vi "IMAQDevice.ProcCases.vi"(0 "i ref in":refnum<vi>, 1 "selector":string, 2 "Data":T1, 3 "call cluster":T2={"Object"="", "Selector"="", "CallType"=enum."synchronous", "Async Object"="", "Async Selector"="", "Data Descriptor"="", "Data"=[], "Error #"=0, "Expire"=0}, 5 "error in (no error)":errorcluster) -> (14 "i ref out":refnum<vi>, 17 "answer cluster":T2={"Object"="", "Selector"="", "CallType"=enum."synchronous", "Async Object"="", "Async Selector"="", "Data Descriptor"="", "Data"=[], "Error #"=0, "Expire"=0}, 19 "error out":errorcluster)   [LabVIEW 2014, in "IMAQDevice.lvlib"]
doc: "This method is called by a process from within the default case in the event loop. The methods of a class that are linked to events will be called from THIS method. Add your code here."
uses:
  IMAQDevice.lvlib
  CSCore/CSApplicationBaseClasses/DeviceBase/DeviceBase.lvlib
  CSCore/BaseProcess/BaseProcess.lvlib
  CSCore/CSSystem/CoreLib/CoreLib.lvlib
  CSCore/CSSystem/CoreLib/CoreLib.string 2 byte array.vi
  CSCore/CSSystem/CoreLib/CoreLib.byte array 2 short.vi
  CSCore/CSSystem/CoreLib/CoreLib.byte array 2 int.vi
  CSCore/CSSystem/CoreLib/CoreLib.int 2 byte array.vi
  CSCore/CSSystem/CoreLib/CoreLib.double 2 byte array.vi
  CSCore/BaseProcess/BaseProcess.descriptor string definition.ctl
  CSlibraries-extern/DimLVEvent/LVDimInterface/LVDimInterface.lvlib
  CSCore/CSSystem/CoreDefs/CoreDefs.call_type.ctl
  CSCore/CSSystem/CoreDefs/CoreDefs.rawDataType.ctl
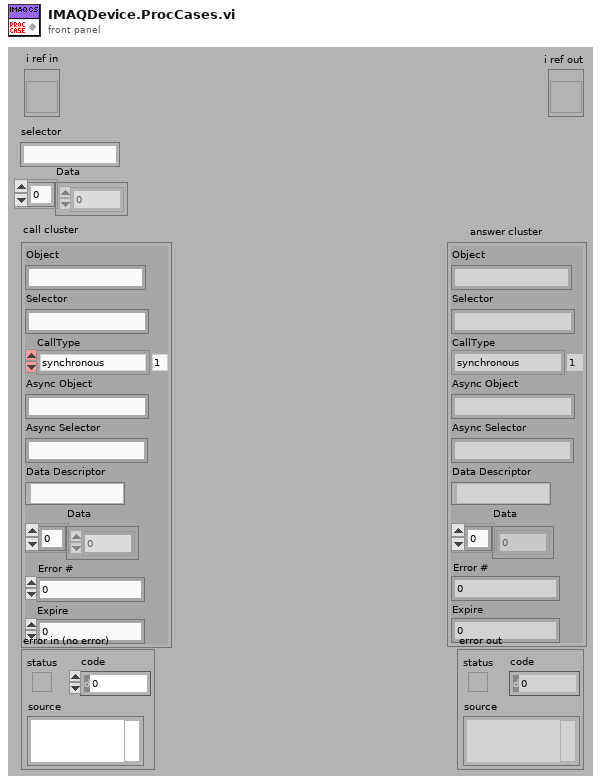
[diagram p1: front panel]
types:
  T1 = typedef "CoreDefs.rawDataType.ctl" = i8[]
  T2 = typedef "CoreDefs.call_type.ctl" = cluster{"Object":string, "Selector":string, "CallType":enum16{"simple", "synchronous", "asynchronous"}, "Async Object":string, "Async Selector":string, "Data Descriptor":T3, "Data":T1, "Error #":i32, "Expire":u32}
  T3 = typedef "BaseProcess.lvlib/BaseProcess.descriptor string definition.ctl" = string
  T4 = typedef "IMAQDevice.lvlib/IMAQDevice.i attribute.ctl" = cluster{"HGF_IMAQ.lvlib:HGF_IMAQDevice.lvclass":refnum<class "HGF_IMAQDevice.lvclass">, "Image":T5, "TimeStampID":i32, "Image IDs":i32[], "NumberOfImagesID":i32, "JPEG?":bool, "JPEGID":i32, "JPEG_ImageID":i32, "TriggerModeID":i32, "OffsetFromLeft":i32, "OffsetFromTop":i32, "HorizontalPixelPerMm":dbl, "VerticalPixelPerMm":dbl, "Grid":cluster{"1":cluster{i32, i32}, "2":cluster{i32, i32}, "3":cluster{i32, i32}, "4":cluster{i32, i32}}, "GridR":cluster{"1":cluster{dbl, dbl}, "2":cluster{dbl, dbl}, "3":cluster{dbl, dbl}, "4":cluster{dbl, dbl}}, "CameraTypeID":i32, "CameraInfos":cluster{"Camera Name-Array":string[], "own Camera Type":string}, "TakeMeasurement?":bool, "TriggerArmedID":i32, "Mirroring":i16, "Rotation":dbl}
  T5 = typedef "IMAQ Image.ctl" = refnum<image>
  T6 = cluster{"1":cluster{i32, i32}, "2":cluster{i32, i32}, "3":cluster{i32, i32}, "4":cluster{i32, i32}}
  T7 = cluster{"1":cluster{dbl, dbl}, "2":cluster{dbl, dbl}, "3":cluster{dbl, dbl}, "4":cluster{dbl, dbl}}
  T8 = cluster{"Grid":cluster{"1":cluster{i32, i32}, "2":cluster{i32, i32}, "3":cluster{i32, i32}, "4":cluster{i32, i32}}, "GridR":cluster{"1":cluster{dbl, dbl}, "2":cluster{dbl, dbl}, "3":cluster{dbl, dbl}, "4":cluster{dbl, dbl}}}
  T9 = cluster{"Camera Name-Array":string[], "own Camera Type":string}
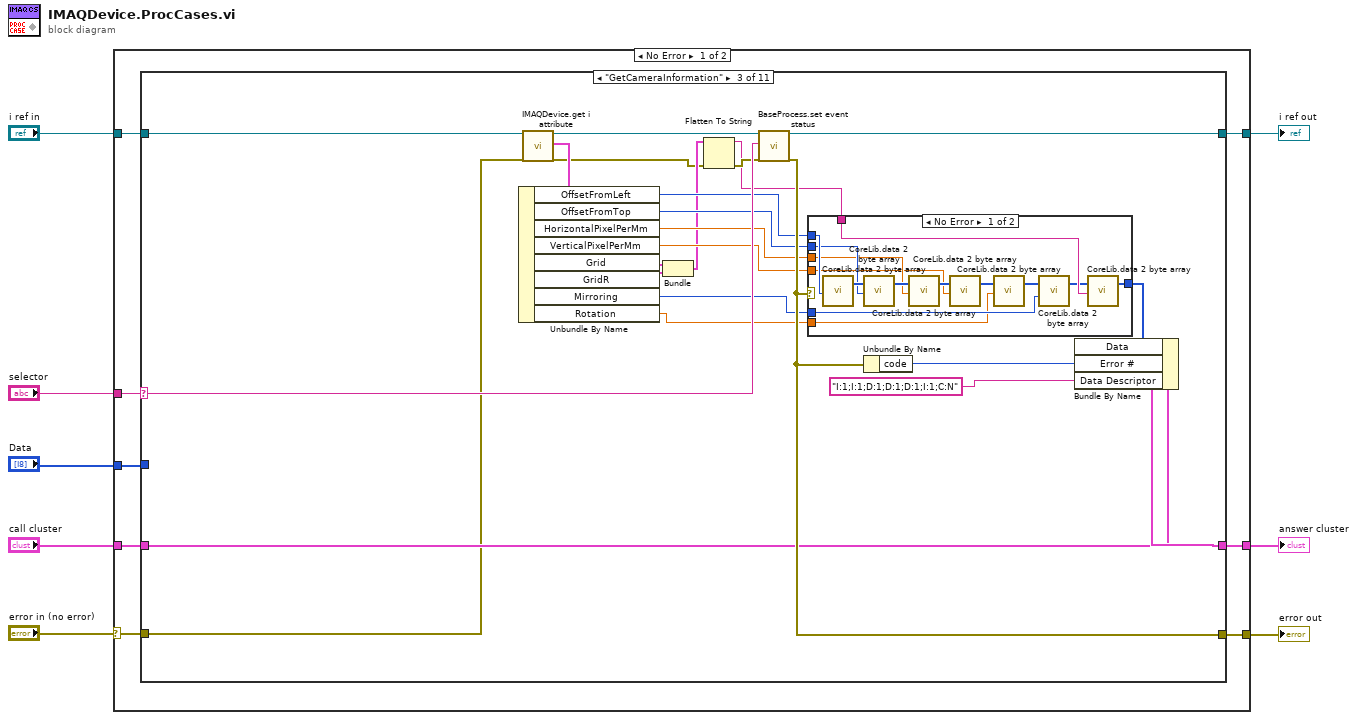
[diagram p0: block diagram]
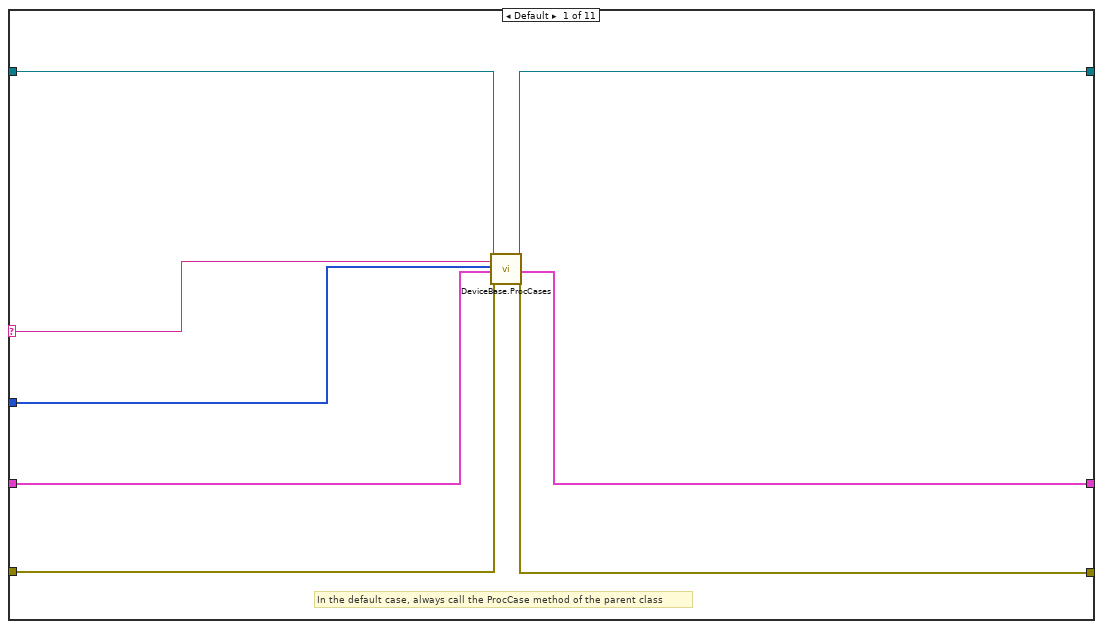
[diagram p2: hidden frame]
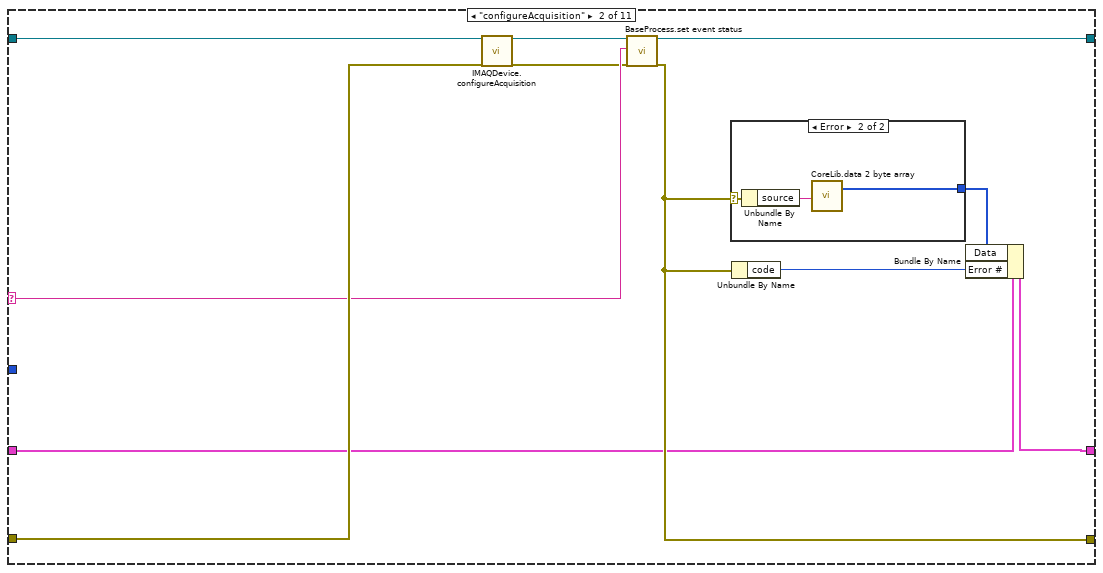
[diagram p3: hidden frame]
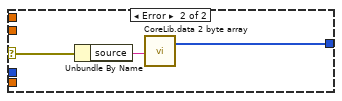
[diagram p5: hidden frame]
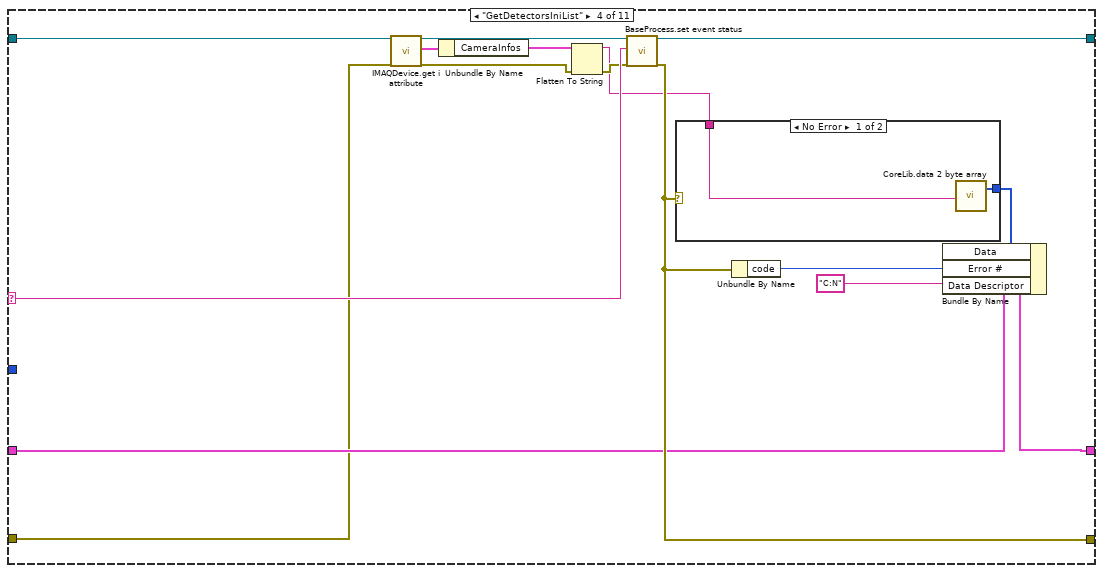
[diagram p6: hidden frame]
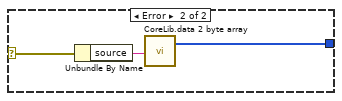
[diagram p7: hidden frame]
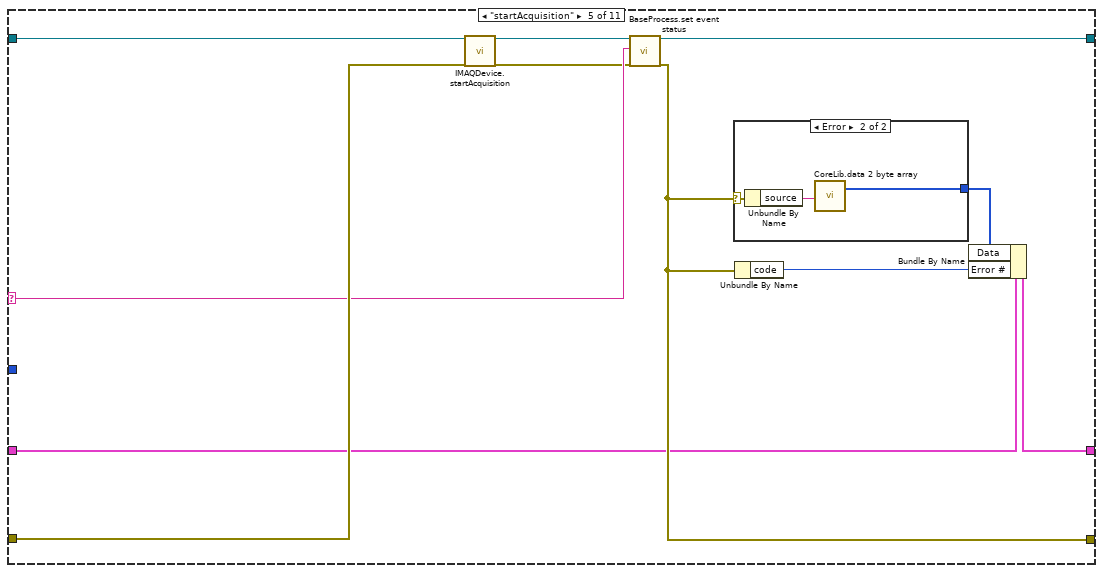
[diagram p8: hidden frame]
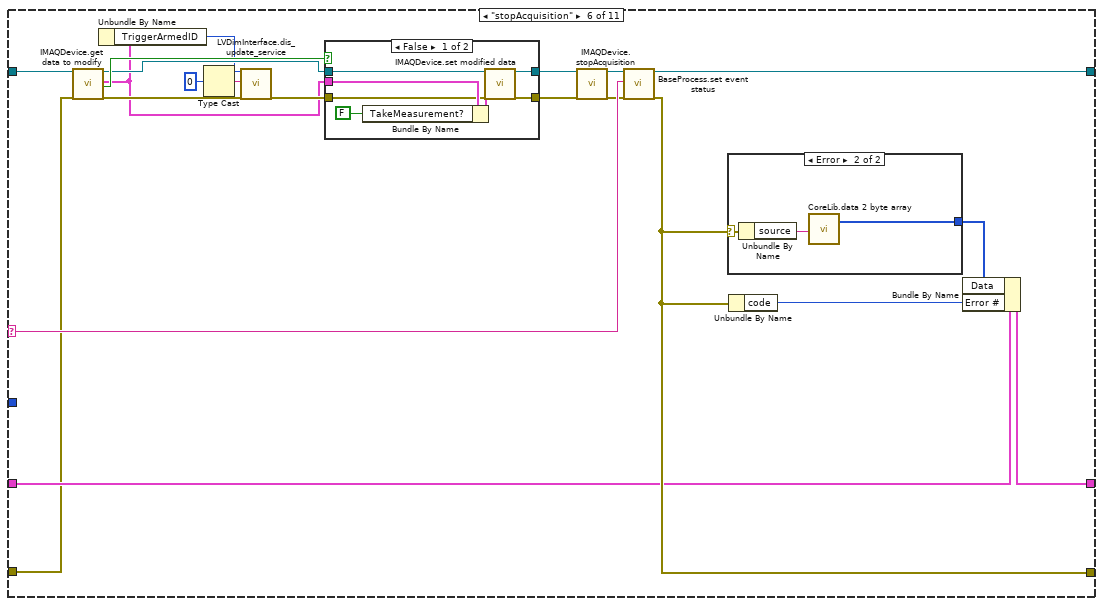
[diagram p10: hidden frame]
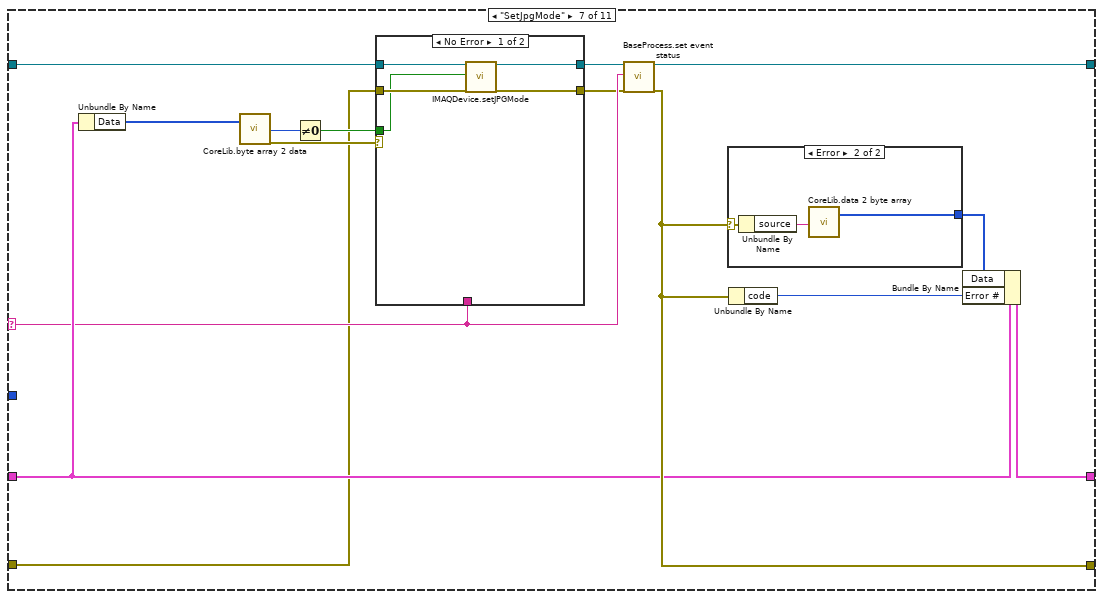
[diagram p13: hidden frame]
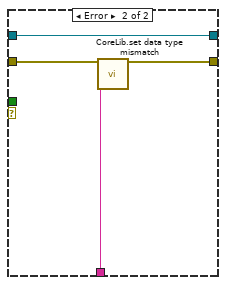
[diagram p14: hidden frame]
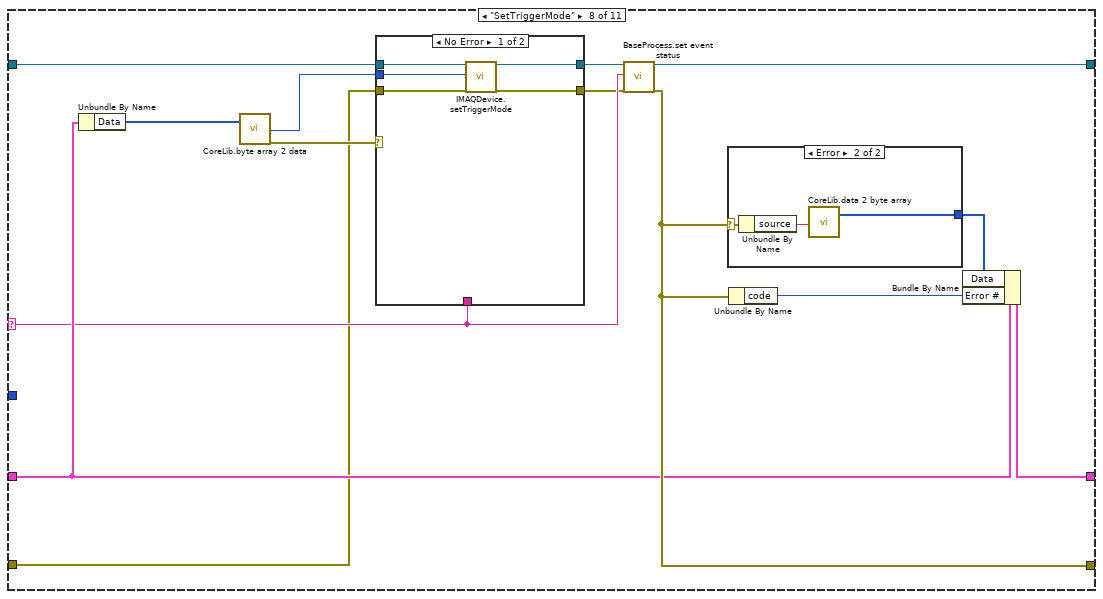
[diagram p16: hidden frame]
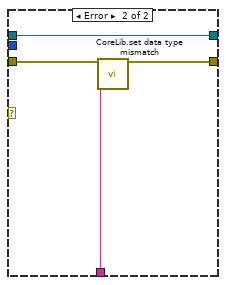
[diagram p17: hidden frame]
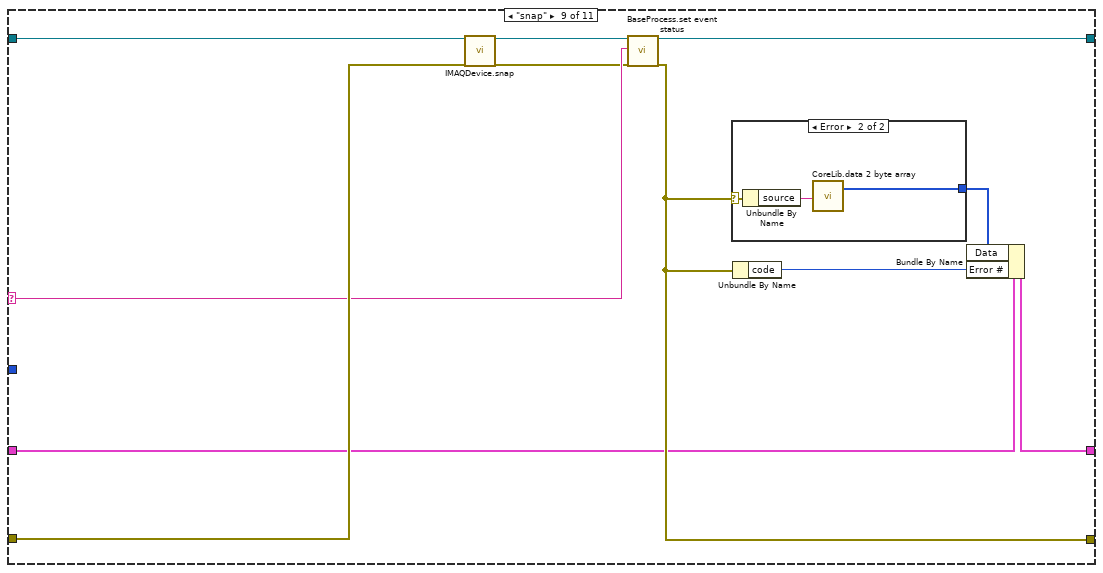
[diagram p19: hidden frame]
diagram:
  n1 = case shown="No Error" "error in (no error)" {
    selector: "error in (no error)" -> [w9 w260]
    tunnel: "selector" -> [w16 _]
    tunnel: [w15 w261] -> w7
    tunnel: "Data" -> [w14 _]
    tunnel: "call cluster" -> [w13 w261]
    tunnel: "i ref in" -> [w12 w262]
    tunnel: [w11 w262] -> w3
    tunnel: [w10 w260] -> w2
    frame No Error {
      n2 = case shown="\"GetCameraInformation\"" w16 {
        selector: w16 -> [w19 w31 w60 w93 w107 w133 w154 w181 w207 w231 w252]
        tunnel: w14 -> [w17 _ _ _ _ _ _ _ _ _ _]
        tunnel: w12 -> [w18 w35 w53 w86 w111 w125 w150 w178 w211 w226 w256]
        tunnel: [w24 w29 w59 w92 w102 w128 w158 w184 w202 w230 w249] -> w11
        tunnel: w13 -> [w20 w25 w56 w89 w103 w129 w155 w182 w203 w227 w246]
        tunnel: [w21 w26 w57 w90 w104 w130 w159 w185 w204 w228 w247] -> w15
        tunnel: w9 -> [w23 w34 w55 w88 w110 w123 w151 w179 w210 w225 w255]
        tunnel: [w22 w27 w58 w91 w105 w131 w160 w186 w205 w229 w248] -> w10
        frame Default {
          # "In the default case, always call the ProcCase method of the parent class"
          n3 = call "DeviceBase.ProcCases.vi"("i ref in"=w18, "selector"=w19, "Data"=w17, "call cluster"=w20, "error in (no error)"=w23) -> ("i ref out"=w24:refnum<vi>, "answer cluster"=w21:T2, "error out"=w22:errorcluster)  [unwired: 12 in]
        }
        frame "configureAcquisition" {
          n4 = call "IMAQDevice.configureAcquisition.vi"("i ref in"=w35, "error in (no error)"=w34) -> ("i ref out"=w28:refnum<vi>, "error out"=w30:errorcluster)  [unwired: 16 in]
          n5 = call "BaseProcess.set event status.vi"("i ref in"=w28, "EventStatus"=w31, "error in (no error)"=w30) -> ("i ref out"=w29:refnum<vi>, "error out"=w27:errorcluster)  [unwired: 14 in, 1 out]
          n6 = case shown="Error" w27 {
            selector: w27 -> [_ w38]
            tunnel: [_ w36] -> w32
            frame No Error {
            }
            frame Error {
              n7 = Unbundle By Name(w38) -> ("source"=w37:string)
              n8 = call-poly "CoreLib.data 2 byte array.vi"("string"=w37) -> ("byteArray out"=w36:T1)  [unwired: 18 in]
            }
          }
          n9 = Unbundle By Name(w27) -> ("code"=w33:i32)
          n10 = Bundle By Name(cluster=w25, "Data"=w32, "Error #"=w33) -> (w26:T2)
        }
        frame "GetCameraInformation" {
          n11 = call "IMAQDevice.get i attribute.vi"("i ref in"=w53, "error in (no error)"=w55) -> ("i ref out"=w54:refnum<vi>, "i attribute"=w52:T4, "error out"=w44:errorcluster)  [unwired: 15 in]
          n12 = Unbundle By Name(w52) -> ("OffsetFromLeft"=w51:i32, "OffsetFromTop"=w50:i32, "HorizontalPixelPerMm"=w49:dbl, "VerticalPixelPerMm"=w48:dbl, "Grid"=w47:T6, "GridR"=w46:T7, "Mirroring"=w40:i16, "Rotation"=w39:dbl)
          n13 = Bundle("Grid"=w47, "GridR"=w46) -> (w45:T8)  [unwired: 1 in]
          n14 = Flatten To String(anything=w45, error in (no error)=w44) -> (data string=w42:string, error out=w43:errorcluster)  [unwired: 2 in, 1 out]
          n15 = call "BaseProcess.set event status.vi"("i ref in"=w54, "EventStatus"=w60, "error in (no error)"=w43) -> ("i ref out"=w59:refnum<vi>, "error out"=w58:errorcluster)  [unwired: 14 in, 1 out]
          n16 = case shown="No Error" w58 {
            selector: w58 -> [_ w79]
            tunnel: [w69 w77] -> w61
            tunnel: w51 -> [w76 _]
            tunnel: w50 -> [w74 _]
            tunnel: w49 -> [w71 _]
            tunnel: w48 -> [w70 _]
            tunnel: w42 -> [w68 _]
            tunnel: w40 -> [w66 _]
            tunnel: w39 -> [w63 _]
            frame No Error {
              n17 = call-poly "CoreLib.data 2 byte array.vi"("i32"=w76) -> ("byteArray out"=w75:T1)  [unwired: 18 in]
              n18 = call-poly "CoreLib.data 2 byte array.vi"("byteArray"=w75, "i32"=w74) -> ("byteArray out"=w73:T1)  [unwired: 17 in]
              n19 = call-poly "CoreLib.data 2 byte array.vi"("byteArray"=w73, "f64"=w71) -> ("byteArray out"=w72:T1)  [unwired: 17 in]
              n20 = call-poly "CoreLib.data 2 byte array.vi"("byteArray"=w72, "f64"=w70) -> ("byteArray out"=w65:T1)  [unwired: 17 in]
              n21 = call-poly "CoreLib.data 2 byte array.vi"("byteArray"=w65, "f64"=w63) -> ("byteArray out"=w64:T1)  [unwired: 17 in]
              n22 = call-poly "CoreLib.data 2 byte array.vi"("byteArray"=w64, "i32"=w66) -> ("byteArray out"=w67:T1)  [unwired: 17 in]
              n23 = call-poly "CoreLib.data 2 byte array.vi"("byteArray"=w67, "string"=w68) -> ("byteArray out"=w69:T1)  [unwired: 17 in]
            }
            frame Error {
              n24 = Unbundle By Name(w79) -> ("source"=w78:string)
              n25 = call-poly "CoreLib.data 2 byte array.vi"("string"=w78) -> ("byteArray out"=w77:T1)  [unwired: 18 in]
            }
          }
          n26 = Unbundle By Name(w58) -> ("code"=w62:i32)
          n27 = Bundle By Name(cluster=w56, "Data"=w61, "Error #"=w62, "Data Descriptor"=T3 "I:1;I:1;D:1;D:1;D:1;I:1;C:N") -> (w57:T2)
        }
        frame "GetDetectorsIniList" {
          n28 = call "IMAQDevice.get i attribute.vi"("i ref in"=w86, "error in (no error)"=w88) -> ("i ref out"=w87:refnum<vi>, "i attribute"=w85:T4, "error out"=w84:errorcluster)  [unwired: 15 in]
          n29 = Unbundle By Name(w85) -> ("CameraInfos"=w80:T9)
          n30 = Flatten To String(anything=w80, error in (no error)=w84) -> (data string=w82:string, error out=w83:errorcluster)  [unwired: 2 in, 1 out]
          n31 = call "BaseProcess.set event status.vi"("i ref in"=w87, "EventStatus"=w93, "error in (no error)"=w83) -> ("i ref out"=w92:refnum<vi>, "error out"=w91:errorcluster)  [unwired: 14 in, 1 out]
          n32 = case shown="No Error" w91 {
            selector: w91 -> [_ w100]
            tunnel: [w97 w98] -> w94
            tunnel: w82 -> [w96 _]
            frame No Error {
              n33 = call-poly "CoreLib.data 2 byte array.vi"("string"=w96) -> ("byteArray out"=w97:T1)  [unwired: 18 in]
            }
            frame Error {
              n34 = Unbundle By Name(w100) -> ("source"=w99:string)
              n35 = call-poly "CoreLib.data 2 byte array.vi"("string"=w99) -> ("byteArray out"=w98:T1)  [unwired: 18 in]
            }
          }
          n36 = Unbundle By Name(w91) -> ("code"=w95:i32)
          n37 = Bundle By Name(cluster=w89, "Data"=w94, "Error #"=w95, "Data Descriptor"=T3 "C:N") -> (w90:T2)
        }
        frame "startAcquisition" {
          n38 = call "IMAQDevice.startAcquisition.vi"("i ref in"=w111, "error in (no error)"=w110) -> ("i ref out"=w101:refnum<vi>, "error out"=w106:errorcluster)  [unwired: 16 in]
          n39 = call "BaseProcess.set event status.vi"("i ref in"=w101, "EventStatus"=w107, "error in (no error)"=w106) -> ("i ref out"=w102:refnum<vi>, "error out"=w105:errorcluster)  [unwired: 14 in, 1 out]
          n40 = case shown="Error" w105 {
            selector: w105 -> [_ w114]
            tunnel: [_ w112] -> w108
            frame No Error {
            }
            frame Error {
              n41 = Unbundle By Name(w114) -> ("source"=w113:string)
              n42 = call-poly "CoreLib.data 2 byte array.vi"("string"=w113) -> ("byteArray out"=w112:T1)  [unwired: 18 in]
            }
          }
          n43 = Unbundle By Name(w105) -> ("code"=w109:i32)
          n44 = Bundle By Name(cluster=w103, "Data"=w108, "Error #"=w109) -> (w104:T2)
        }
        frame "stopAcquisition" {
          n45 = call "IMAQDevice.get data to modify.vi"("i ref in"=w125, "error in (no error)"=w123) -> ("i ref out"=w119:refnum<vi>, "i attribute"=w116:T4, "timed out"=w126:bool, "error out"=w121:errorcluster)  [unwired: 14 in]
          n46 = Unbundle By Name(w116) -> ("TriggerArmedID"=w115:i32)
          n47 = Type Cast(x=0) -> (*(type *) &x=w118:string)  [unwired: 1 in]
          n48 = call "LVDimInterface.dis_update_service.vi"("my_serviceID"=w115, "data"=w118, "error in (no error)"=w121) -> ("error out"=w120:errorcluster)  [unwired: 14 in, 2 out]
          n49 = case shown="False" w126 {
            tunnel: w116 -> [w142 _]
            tunnel: w120 -> [w141 w143]
            tunnel: [w140 w143] -> w122
            tunnel: [w139 w144] -> w124
            tunnel: w119 -> [w137 w144]
            frame False {
              n50 = Bundle By Name(cluster=w142, "TakeMeasurement?"=FALSE) -> (w138:T4)
              n51 = call "IMAQDevice.set modified data.vi"("i ref in"=w137, "i attribute"=w138, "error in (no error)"=w141) -> ("i ref out"=w139:refnum<vi>, "error out"=w140:errorcluster)  [unwired: 15 in]
            }
            frame True {
            }
          }
          n52 = call "IMAQDevice.stopAcquisition.vi"("i ref in"=w124, "error in (no error)"=w122) -> ("i ref out"=w127:refnum<vi>, "error out"=w132:errorcluster)  [unwired: 16 in]
          n53 = call "BaseProcess.set event status.vi"("i ref in"=w127, "EventStatus"=w133, "error in (no error)"=w132) -> ("i ref out"=w128:refnum<vi>, "error out"=w131:errorcluster)  [unwired: 14 in, 1 out]
          n54 = case shown="Error" w131 {
            selector: w131 -> [_ w147]
            tunnel: [_ w145] -> w134
            frame No Error {
            }
            frame Error {
              n55 = Unbundle By Name(w147) -> ("source"=w146:string)
              n56 = call-poly "CoreLib.data 2 byte array.vi"("string"=w146) -> ("byteArray out"=w145:T1)  [unwired: 18 in]
            }
          }
          n57 = Unbundle By Name(w131) -> ("code"=w135:i32)
          n58 = Bundle By Name(cluster=w129, "Data"=w134, "Error #"=w135) -> (w130:T2)
        }
        frame "SetJpgMode" {
          n59 = Unbundle By Name(w155) -> ("Data"=w157:T1)
          n60 = call-poly "CoreLib.byte array 2 data.vi"("byteArray"=w157) -> ("i16"=w156:i16, "error out"=w153:errorcluster)  [unwired: 16 in, 1 out]
          n61 = Not Equal To 0?(x=w156) -> (x != 0?=w152:bool)
          n62 = case shown="No Error" w153 {
            tunnel: [w166 w168] -> w149
            tunnel: w150 -> [w167 w168]
            tunnel: [w164 w171] -> w148
            tunnel: w154 -> [_ w170]
            tunnel: w152 -> [w163 _]
            tunnel: w151 -> [w165 w169]
            frame No Error {
              n63 = call "IMAQDevice.setJPGMode.vi"("i ref in"=w167, "JPEG Mode?"=w163, "error in (no error)"=w165) -> ("i ref out"=w166:refnum<vi>, "error out"=w164:errorcluster)  [unwired: 15 in]
            }
            frame Error {
              n64 = call "CoreLib.set data type mismatch.vi"("error in (no error)"=w169, "error source"=w170) -> ("error out"=w171:errorcluster)  [unwired: 17 in]
            }
          }
          n65 = call "BaseProcess.set event status.vi"("i ref in"=w149, "EventStatus"=w154, "error in (no error)"=w148) -> ("i ref out"=w158:refnum<vi>, "error out"=w160:errorcluster)  [unwired: 14 in, 1 out]
          n66 = case shown="Error" w160 {
            selector: w160 -> [_ w174]
            tunnel: [_ w172] -> w161
            frame No Error {
            }
            frame Error {
              n67 = Unbundle By Name(w174) -> ("source"=w173:string)
              n68 = call-poly "CoreLib.data 2 byte array.vi"("string"=w173) -> ("byteArray out"=w172:T1)  [unwired: 18 in]
            }
          }
          n69 = Unbundle By Name(w160) -> ("code"=w162:i32)
          n70 = Bundle By Name(cluster=w155, "Data"=w161, "Error #"=w162) -> (w159:T2)
        }
        frame "SetTriggerMode" {
          n71 = Unbundle By Name(w182) -> ("Data"=w183:T1)
          n72 = call-poly "CoreLib.byte array 2 data.vi"("byteArray"=w183) -> ("i32"=w175:i32, "error out"=w180:errorcluster)  [unwired: 16 in, 1 out]
          n73 = case shown="No Error" w180 {
            tunnel: [w192 w194] -> w177
            tunnel: w178 -> [w193 w194]
            tunnel: [w190 w197] -> w176
            tunnel: w181 -> [_ w196]
            tunnel: w179 -> [w191 w195]
            tunnel: w175 -> [w189 _]
            frame No Error {
              n74 = call "IMAQDevice.setTriggerMode.vi"("i ref in"=w193, "TriggerMode"=w189, "error in (no error)"=w191) -> ("i ref out"=w192:refnum<vi>, "error out"=w190:errorcluster)  [unwired: 15 in]
            }
            frame Error {
              n75 = call "CoreLib.set data type mismatch.vi"("error in (no error)"=w195, "error source"=w196) -> ("error out"=w197:errorcluster)  [unwired: 17 in]
            }
          }
          n76 = call "BaseProcess.set event status.vi"("i ref in"=w177, "EventStatus"=w181, "error in (no error)"=w176) -> ("i ref out"=w184:refnum<vi>, "error out"=w186:errorcluster)  [unwired: 14 in, 1 out]
          n77 = case shown="Error" w186 {
            selector: w186 -> [_ w200]
            tunnel: [_ w198] -> w187
            frame No Error {
            }
            frame Error {
              n78 = Unbundle By Name(w200) -> ("source"=w199:string)
              n79 = call-poly "CoreLib.data 2 byte array.vi"("string"=w199) -> ("byteArray out"=w198:T1)  [unwired: 18 in]
            }
          }
          n80 = Unbundle By Name(w186) -> ("code"=w188:i32)
          n81 = Bundle By Name(cluster=w182, "Data"=w187, "Error #"=w188) -> (w185:T2)
        }
        frame "snap" {
          n82 = call "IMAQDevice.snap.vi"("i ref in"=w211, "error in (no error)"=w210) -> ("i ref out"=w201:refnum<vi>, "error out"=w206:errorcluster)  [unwired: 16 in]
          n83 = call "BaseProcess.set event status.vi"("i ref in"=w201, "EventStatus"=w207, "error in (no error)"=w206) -> ("i ref out"=w202:refnum<vi>, "error out"=w205:errorcluster)  [unwired: 14 in, 1 out]
          n84 = case shown="Error" w205 {
            selector: w205 -> [_ w214]
            tunnel: [_ w212] -> w208
            frame No Error {
            }
            frame Error {
              n85 = Unbundle By Name(w214) -> ("source"=w213:string)
              n86 = call-poly "CoreLib.data 2 byte array.vi"("string"=w213) -> ("byteArray out"=w212:T1)  [unwired: 18 in]
            }
          }
          n87 = Unbundle By Name(w205) -> ("code"=w209:i32)
          n88 = Bundle By Name(cluster=w203, "Data"=w208, "Error #"=w209) -> (w204:T2)
        }
        frame "snap_and_publish" {
          n89 = call "IMAQDevice.get data to modify.vi"("i ref in"=w226, "error in (no error)"=w225) -> ("i ref out"=w219:refnum<vi>, "i attribute"=w216:T4, "timed out"=w222:bool, "error out"=w221:errorcluster)  [unwired: 14 in]
          n90 = Unbundle By Name(w216) -> ("TriggerArmedID"=w215:i32)
          n91 = Type Cast(x=1) -> (*(type *) &x=w218:string)  [unwired: 1 in]
          n92 = call "LVDimInterface.dis_update_service.vi"("my_serviceID"=w215, "data"=w218, "error in (no error)"=w221) -> ("error out"=w220:errorcluster)  [unwired: 14 in, 2 out]
          n93 = case shown="False" w222 {
            tunnel: w216 -> [w240 _]
            tunnel: w220 -> [w239 w241]
            tunnel: [w238 w241] -> w224
            tunnel: [w237 w242] -> w223
            tunnel: w219 -> [w235 w242]
            frame False {
              n94 = Bundle By Name(cluster=w240, "TakeMeasurement?"=TRUE) -> (w236:T4)
              n95 = call "IMAQDevice.set modified data.vi"("i ref in"=w235, "i attribute"=w236, "error in (no error)"=w239) -> ("i ref out"=w237:refnum<vi>, "error out"=w238:errorcluster)  [unwired: 15 in]
            }
            frame True {
            }
          }
          n96 = call "BaseProcess.set event status.vi"("i ref in"=w223, "EventStatus"=w231, "error in (no error)"=w224) -> ("i ref out"=w230:refnum<vi>, "error out"=w229:errorcluster)  [unwired: 14 in, 1 out]
          n97 = case shown="Error" w229 {
            selector: w229 -> [_ w245]
            tunnel: [_ w243] -> w232
            frame No Error {
            }
            frame Error {
              n98 = Unbundle By Name(w245) -> ("source"=w244:string)
              n99 = call-poly "CoreLib.data 2 byte array.vi"("string"=w244) -> ("byteArray out"=w243:T1)  [unwired: 18 in]
            }
          }
          n100 = Unbundle By Name(w229) -> ("code"=w233:i32)
          n101 = Bundle By Name(cluster=w227, "Data"=w232, "Error #"=w233) -> (w228:T2)
        }
        frame "getImage" {
          n102 = call "IMAQDevice.getImage.vi"("i ref in"=w256, "error in (no error)"=w255) -> ("i ref out"=w250:refnum<vi>, "error out"=w251:errorcluster)  [unwired: 16 in]
          n103 = call "BaseProcess.set event status.vi"("i ref in"=w250, "EventStatus"=w252, "error in (no error)"=w251) -> ("i ref out"=w249:refnum<vi>, "error out"=w248:errorcluster)  [unwired: 14 in, 1 out]
          n104 = case shown="Error" w248 {
            selector: w248 -> [_ w259]
            tunnel: [_ w257] -> w253
            frame No Error {
            }
            frame Error {
              n105 = Unbundle By Name(w259) -> ("source"=w258:string)
              n106 = call-poly "CoreLib.data 2 byte array.vi"("string"=w258) -> ("byteArray out"=w257:T1)  [unwired: 18 in]
            }
          }
          n107 = Unbundle By Name(w248) -> ("code"=w254:i32)
          n108 = Bundle By Name(cluster=w246, "Data"=w253, "Error #"=w254) -> (w247:T2)
        }
      }
    }
    frame Error {
    }
  }
  "answer cluster" <- w7
  "i ref out" <- w3
  "error out" <- w2
